vi "GE 5565PIORC.Registers.INTCSR.Local Interrupt Input Enable.Set.vi"(8 "error in (no error)":errorcluster, 10 "Local Interrupt Input Enable":bool, 11 "GE 5565PIORC in":refnum<class "GE 5565PIORC.lvclass">) -> (0 "error out":errorcluster, 3 "GE 5565PIORC out":refnum<class "GE 5565PIORC.lvclass">)   [LabVIEW 2016, in "GE 5565PIORC.lvclass"]
doc: "Writing a one (1) enables a local interrupt (i.e., RFM interrupts) to assert a host Interrupt."
uses:
  GE 5565PIORC.lvclass
  GE 5565PIORC.Registers.Local Configuration.ctl
  GE 5565PIORC.lvclass/GE 5565PIORC.ctl
  GE 5565PIORC.Registers.Local Configuration.Read (U32).vi
  GE 5565PIORC.Registers.Local Configuration.Write (U32).vi
  Bit Manipulation.Set Bit (U32).vi
  GE 5565PIORC.Registers.Read.vi
  GE 5565PIORC.Registers.Read (U32).vi
  GE 5565PIORC.Registers.Write.vi
  GE 5565PIORC.Registers.Write (U32).vi
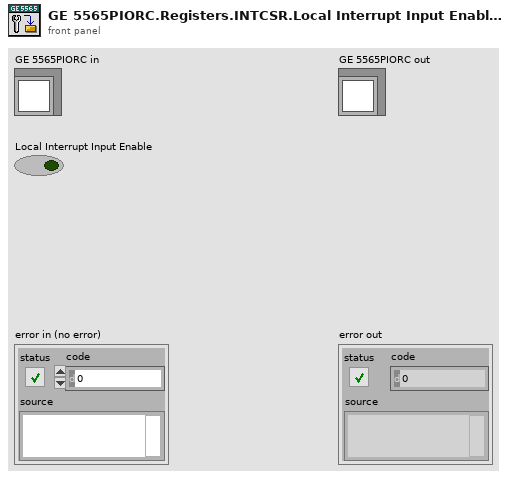
[diagram p1: front panel]
types:
  T1 = typedef "GE 5565PIORC.lvclass/GE 5565PIORC.Registers.Local Configuration.ctl" = u32
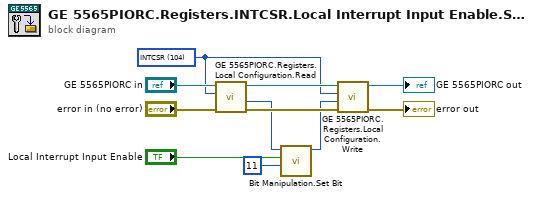
[diagram p0: block diagram]
diagram:
  w5 = T1 104 items=["MARBR"=8, "BIGEND"=12, "INTCSR"=104, "PCIHREV"=116, "DMAMODE0"=128, "DMAPADR0"=132, "DMALADR0"=136, "DMASIZ0"=140, "DMADPR0"=144, "DMACSR0"=168, "DMADAC0"=180, "LAS1RR"=240, "LAS1BA"=244] ("Local Configuration Registers")
  n1 = call-poly "GE 5565PIORC.Registers.Local Configuration.Read.vi"("error in (no error)"="error in (no error)", "Register"=w5, "GE 5565PIORC in"="GE 5565PIORC in") -> ("error out"=w11:errorcluster, "Value"=w4:u32, "GE 5565PIORC out"=w8:refnum<class "GE 5565PIORC.lvclass">)  [unwired: 6 in]
  n2 = call-poly "Bit Manipulation.Set Bit.vi"("bit index"=11, "bit"="Local Interrupt Input Enable", "packed value in"=w4) -> ("packed value out"=w3:u32)  [unwired: 8 in]
  n3 = call-poly "GE 5565PIORC.Registers.Local Configuration.Write.vi"("error in (no error)"=w11, "Value"=w3, "Register"=w5, "GE 5565PIORC in"=w8) -> ("error out"=→"error out":errorcluster, "GE 5565PIORC out"=→"GE 5565PIORC out":refnum<class "GE 5565PIORC.lvclass">)  [unwired: 6 in]
